vi "FlatToRichgrpc_reflection_v1alpha_ErrorResponse.vi"(5 "OutputClusterType":T1, 11 "InputCluster":T2) -> (3 "OutputCluster":T1)   [LabVIEW 2025, in "reflection_server.lvlib"]
uses:
  reflection_server.lvlib
  grpc_reflection_v1alpha_ErrorResponse_Flat.ctl
  grpc_reflection_v1alpha_ErrorResponse.ctl
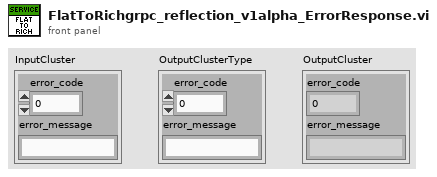
[diagram p1: front panel]
types:
  T1 = typedef "reflection_server.lvlib/grpc_reflection_v1alpha_ErrorResponse.ctl" = cluster{"error_code":i32, "error_message":string}
  T2 = typedef "reflection_server.lvlib/grpc_reflection_v1alpha_ErrorResponse_Flat.ctl" = cluster{"error_code":i32, "error_message":string}
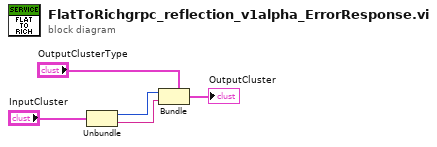
[diagram p0: block diagram]
diagram:
  n1 = Unbundle "Unbundle"("InputCluster") -> ("error_code"=w2:i32, "error_message"=w1:string)
  n2 = Bundle "Bundle"(cluster="OutputClusterType", "error_code"=w2, "error_message"=w1) -> (→"OutputCluster":T1)
